vi "update destination folder.vi"(8 "error in":errorcluster, 11 "Video File in":refnum<class "Video File.lvclass">) -> (0 "error out":errorcluster, 3 "Video File out":refnum<class "Video File.lvclass">)   [LabVIEW 2023, in "File Classes.lvlib" / "Video File.lvclass"]
uses:
  Video File.lvclass
  Video File.lvclass/Video File.ctl
  File/File.lvclass/File.ctl
  File/Accessors/Write destination path.vi
  File/Accessors/Read destination path.vi
  File/Accessors/Read mode.vi
  File/File.lvclass
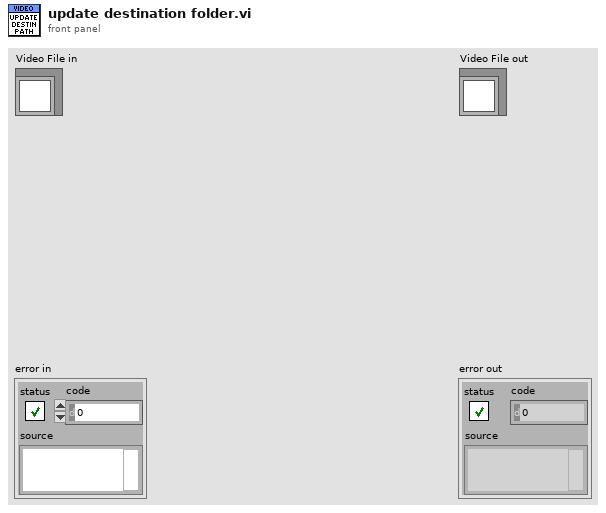
[diagram p1: front panel]
types:
  T1 = typedef "File Classes.lvlib/file operation settings mode.ctl" = enum16{"Copy Files", "Move Files", "Rename Files"}
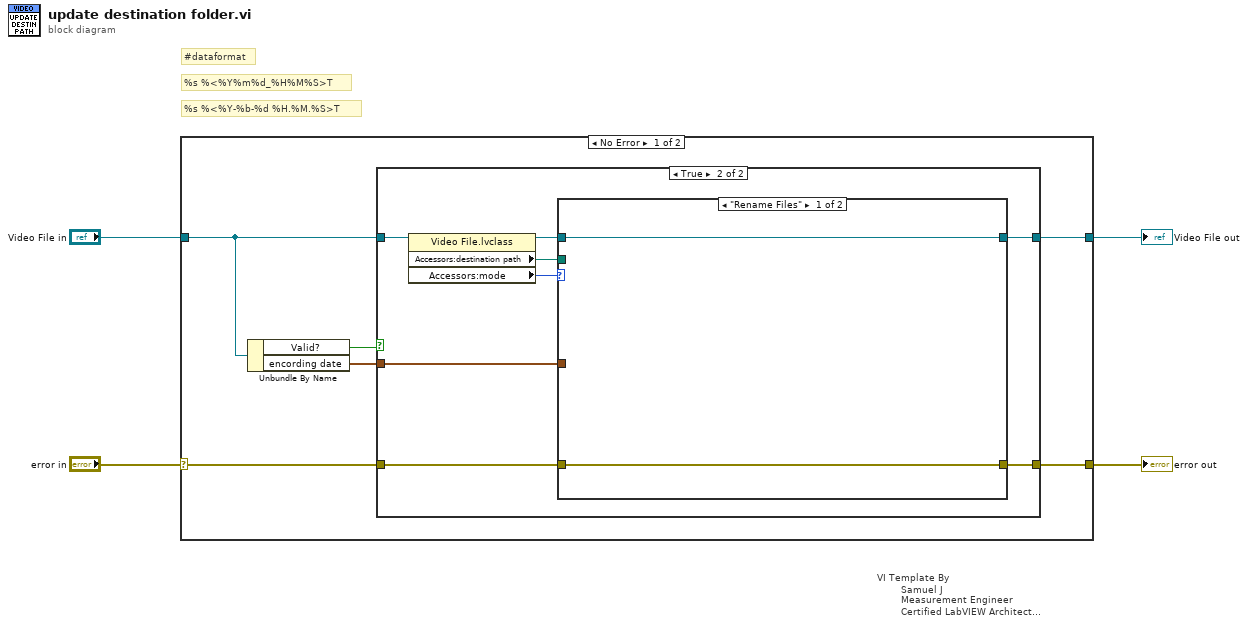
[diagram p0: block diagram]
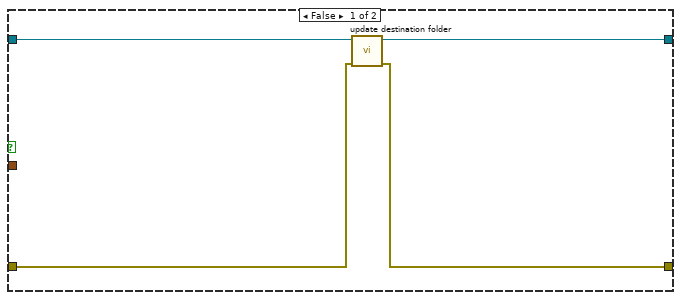
[diagram p2: hidden frame]
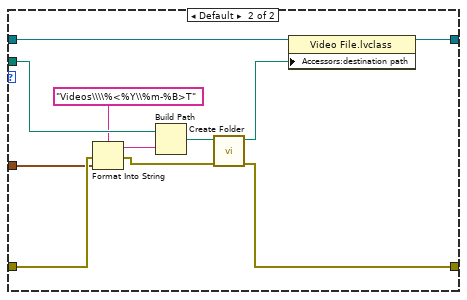
[diagram p3: hidden frame]
diagram:
  # "#dataformat"
  # "%s %<%Y-%b-%d %H.%M.%S>T"
  # "%s %<%Y%m%d_%H%M%S>T"
  n1 = case "VI Template By\n        Samuel J\n        Measurement Engineer\n        Certified LabVIEW Architect\n        Vestas Technology R&D Chennai" shown="No Error" "error in" {
    selector: "error in" -> [w7 w37]
    tunnel: [w8 w37] -> w2
    tunnel: [w10 w36] -> w1
    tunnel: "Video File in" -> [w9 w36]
    frame No Error {
      n2 = Unbundle By Name(w9) -> ("Valid?"=w6:bool, "encording date"=w5:timestamp)
      n3 = case shown="True" w6 {
        tunnel: [w14 w20] -> w10
        tunnel: w9 -> [w13 w22]
        tunnel: [w11 w16] -> w8
        tunnel: w7 -> [w12 w18]
        tunnel: w5 -> [_ w17]
        frame False {
          n4 = call-parent "update destination folder.vi"("error in (no error)"=w12, "File in"=w13) -> ("error out"=w11:errorcluster, "File out"=w14:refnum<class "Video File.lvclass">)  [unwired: 8 in]
        }
        frame True {
          n5 = property class="Video File.lvclass"(reference=w22) -> (reference out=w21:refnum<class "Video File.lvclass">, "Accessors:destination path"=w19:path, "Accessors:mode"=w15:T1)  [unwired: 1 in, 1 out]
          n6 = case shown="\"Rename Files\"" w15 {
            tunnel: w21 -> [w24 w35]
            tunnel: [w24 w34] -> w20
            tunnel: w19 -> [_ w33]
            tunnel: w18 -> [w23 w31]
            tunnel: w17 -> [_ w29]
            tunnel: [w23 w25] -> w16
            frame "Rename Files" {
            }
            frame Default {
              n7 = Format Into String(format string="Videos\\\\%<%Y\\%m-%B>T", error in=w31, w29) -> (resulting string=w32:string, error out=w26:errorcluster)  [unwired: 1 in]
              n8 = Build Path(base path=w33, name or relative path=w32) -> (appended path=w28:path)
              n9 = call <userlib>:"Create Folder.vi"("error in"=w26, "Directory Path"=w28) -> ("error out"=w25:errorcluster, "dup Directory Path"=w27:path)  [unwired: 8 in]
              n10 = property class="Video File.lvclass"(reference=w35, "Accessors:destination path"=w27) -> (reference out=w34:refnum<class "Video File.lvclass">)  [unwired: 1 in, 1 out]
            }
          }
        }
      }
    }
    frame Error {
    }
  }
  "error out" <- w2
  "Video File out" <- w1
